vi "T1T2占空比.vi"() -> ()   [LabVIEW 2020]
uses:
  <vilib>/DAQmx/read.llb/DAQmx Read (Counter 1D DBL 1Chan NSamp).vi
  Global_Variable/Global.vi
  <vilib>/DAQmx/create/channels.llb/DAQmx Create Channel (CI-Period).vi
  <vilib>/DAQmx/configure/timing.llb/DAQmx Timing (Implicit).vi
  <vilib>/DAQmx/miscellaneous.llb/DAQmx Fill In Error Info.vi
  <userlib>/_MGI/1D Array/MGI Average/MGI Average (DBL[]).vi
  <vilib>/DAQmx/create/channels.llb/DAQmx Create Channel (CI-Pulse Width).vi
  <resource>/objmgr/daqmx.rc
panel:
  out "T1 2":dbl
  out "T2 2":dbl
  out "T2":dbl
  out "T2周期":dbl
  out "T1周期":dbl
  out "T1":dbl
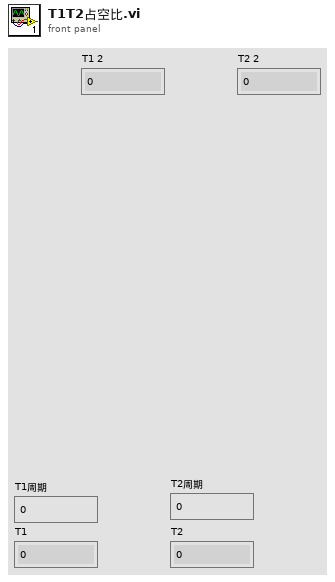
[diagram p1: front panel]
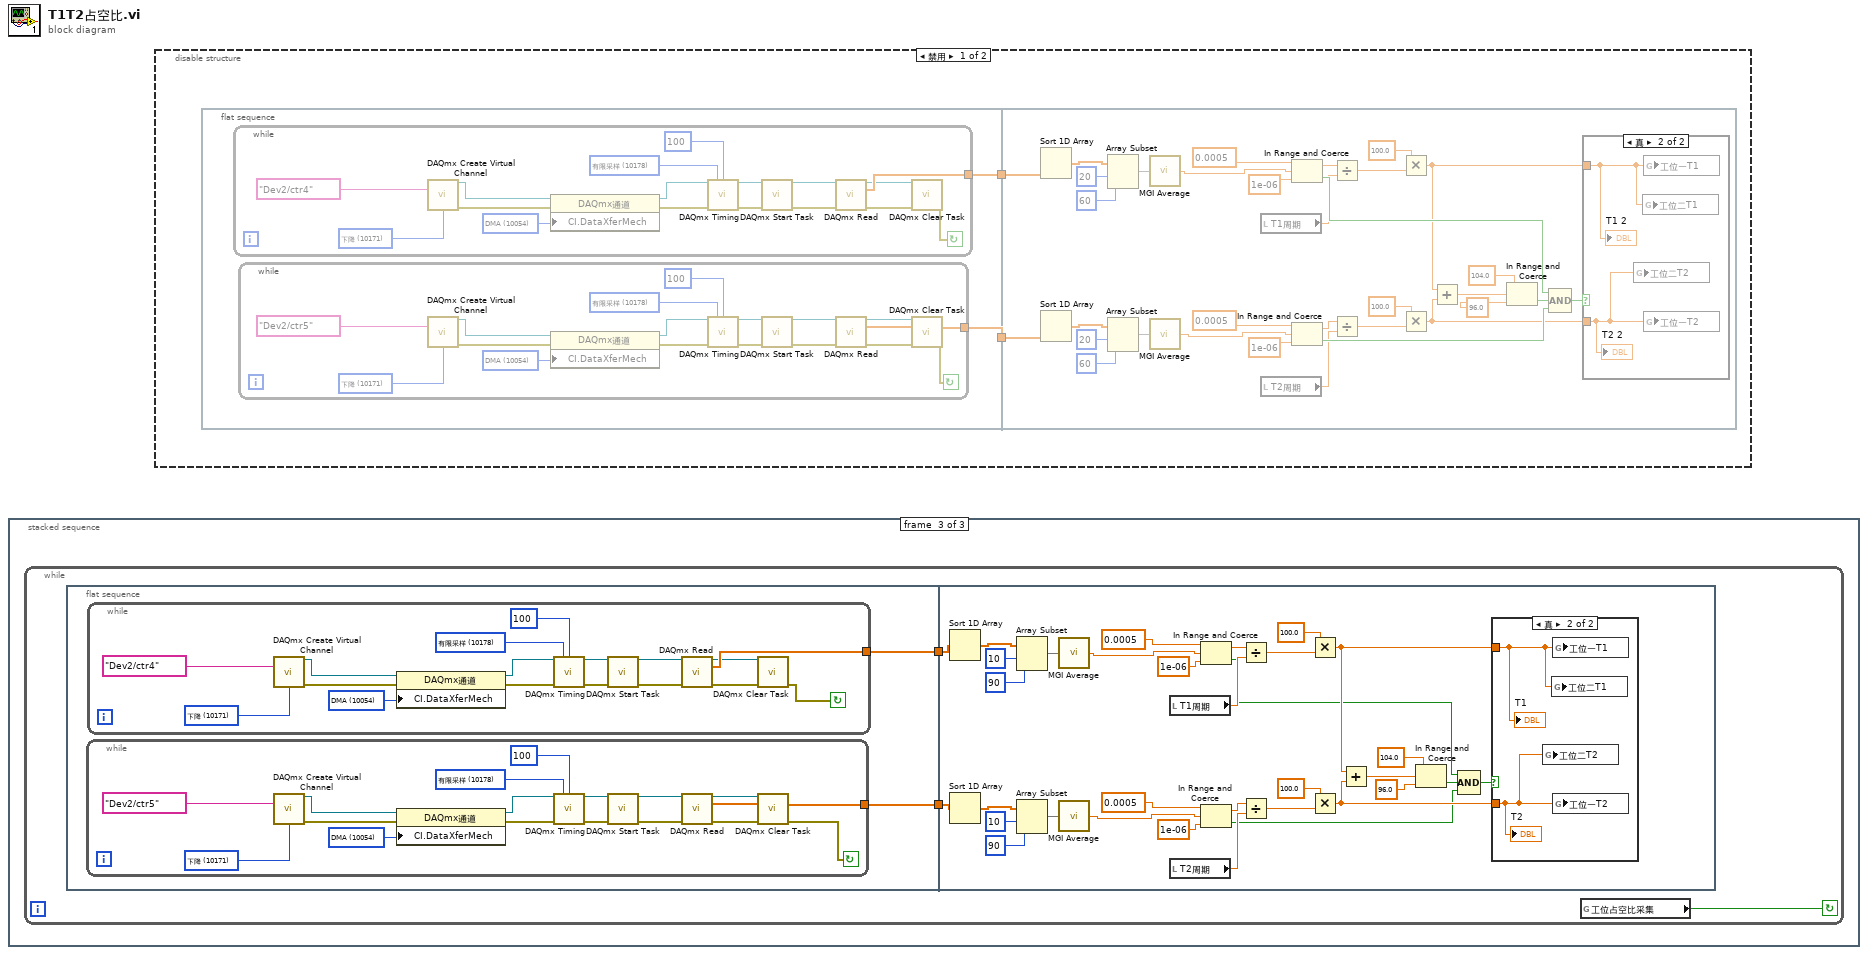
[diagram p0: block diagram]
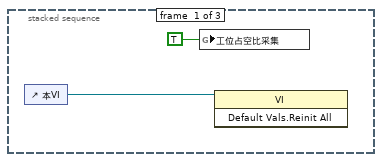
[diagram p4: hidden frame]
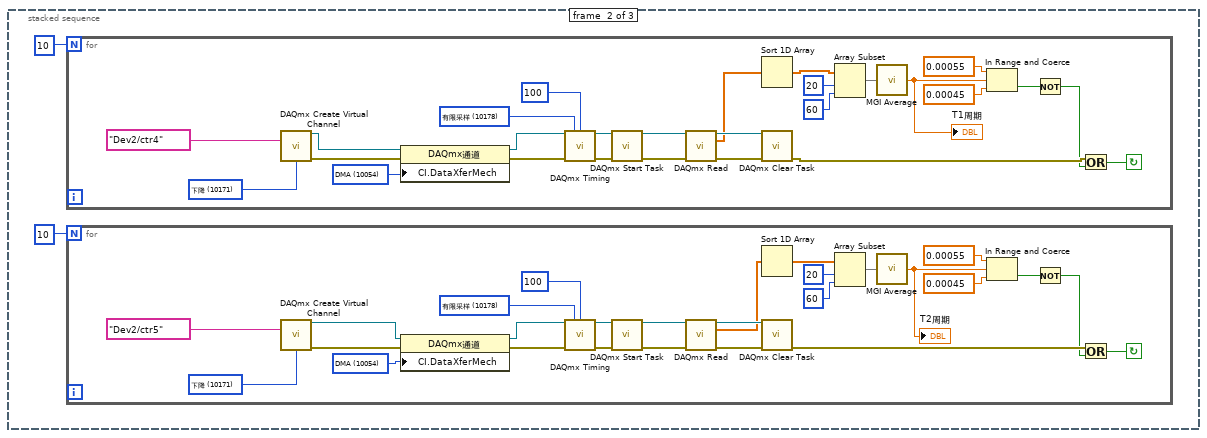
[diagram p5: hidden frame]
diagram:
  n1 = stacked-sequence {
    frame #0 {
      n2 = control-ref of="本VI"() -> (w2:refnum<vi>)
      n3 = global write "Global.vi" "工位占空比采集"(TRUE ("工位一占空比采集")) -> ()
      n4 = invoke class="VI" method="Default Vals.Reinit All"(reference=w2) -> ()  [unwired: 2 in, 3 out]
    }
    frame #1 {
      n5 = for {
        N: 10 -> [_]
        stop <- w32 continue-if-true
        w45 = 10054 items=["DMA"=10054, "中断"=10204, "程序控制I/O"=10264, "USB Bulk"=12590] ("CI.DataXferMech")
        w49 = 10178 items=["有限采样"=10178, "连续采样"=10123, "硬件定时单点"=12522] ("sample mode")
        w58 = 10171 items=["上升"=10280, "下降"=10171] ("starting edge")
        n6 = call-poly <vilib>:"DAQmx Create Virtual Channel.vi"("counter"=tag "Dev2/ctr4", "starting edge"=w58) -> ("task out"=w57:refnum<k21>, "error out"=w47:errorcluster)  [unwired: 12 in]
        n7 = property class="DAQmx通道"(reference=w57, error in=w47, "CI.DataXferMech"=w45) -> (reference out=w48:refnum<k21>, error out=w46:errorcluster)
        n8 = call-poly <vilib>:"DAQmx Timing.vi"("task/channels in"=w48, "sample mode"=w49, "samples per channel"=100, "error in"=w46) -> ("task out"=w56:refnum<k21>, "error out"=w55:errorcluster)  [unwired: 10 in]
        n9 = call <vilib>:"DAQmx Start Task.vi"("task/channels in"=w56, "error in"=w55) -> ("task out"=w54:refnum<k21>, "error out"=w53:errorcluster)  [unwired: 12 in]
        n10 = call-poly <vilib>:"DAQmx Read.vi"("task/channels in"=w54, "error in"=w53) -> ("task out"=w51:refnum<k21>, "data"=w39:dbl[], "error out"=w52:errorcluster)  [unwired: 11 in]
        n11 = Sort 1D Array(array=w39) -> (sorted array=w42:dbl[])
        n12 = call <vilib>:"DAQmx Clear Task.vi"("task in"=w51, "error in"=w52) -> ("error out"=w34:errorcluster)  [unwired: 13 in]
        n13 = Array Subset(array=w42, index=20 ("索引"), length=60 ("长度")) -> (w43:dbl[])
        n14 = call-poly <userlib>:"MGI Average.vi"("Double[]"=w43) -> ("Average"=w38:dbl)  [unwired: 1 in]
        "T1周期" <- w38
        n15 = In Range and Coerce(upper limit=0.00055 ("上限"), x=w38, lower limit=0.00045 ("上限")) -> (In Range?=w35:bool)  [unwired: 1 out]
        n16 = Not(x=w35) -> (.not. x?=w33:bool)
        n17 = Or(x=w34, y=w33) -> (x .or. y?=w32:bool)
      }
      n18 = for {
        N: 10 -> [_]
        stop <- w5 continue-if-true
        w18 = 10054 items=["DMA"=10054, "中断"=10204, "程序控制I/O"=10264, "USB Bulk"=12590] ("CI.DataXferMech")
        w22 = 10178 items=["有限采样"=10178, "连续采样"=10123, "硬件定时单点"=12522] ("sample mode")
        w31 = 10171 items=["上升"=10280, "下降"=10171] ("starting edge")
        n19 = call-poly <vilib>:"DAQmx Create Virtual Channel.vi"("counter"=tag "Dev2/ctr5", "starting edge"=w31) -> ("task out"=w30:refnum<k21>, "error out"=w20:errorcluster)  [unwired: 12 in]
        n20 = property class="DAQmx通道"(reference=w30, error in=w20, "CI.DataXferMech"=w18) -> (reference out=w21:refnum<k21>, error out=w19:errorcluster)
        n21 = call-poly <vilib>:"DAQmx Timing.vi"("task/channels in"=w21, "sample mode"=w22, "samples per channel"=100, "error in"=w19) -> ("task out"=w29:refnum<k21>, "error out"=w28:errorcluster)  [unwired: 10 in]
        n22 = call <vilib>:"DAQmx Start Task.vi"("task/channels in"=w29, "error in"=w28) -> ("task out"=w27:refnum<k21>, "error out"=w26:errorcluster)  [unwired: 12 in]
        n23 = call-poly <vilib>:"DAQmx Read.vi"("task/channels in"=w27, "error in"=w26) -> ("task out"=w24:refnum<k21>, "data"=w12:dbl[], "error out"=w25:errorcluster)  [unwired: 11 in]
        n24 = Sort 1D Array(array=w12) -> (sorted array=w16:dbl[])
        n25 = call <vilib>:"DAQmx Clear Task.vi"("task in"=w24, "error in"=w25) -> ("error out"=w8:errorcluster)  [unwired: 13 in]
        n26 = Array Subset(array=w16, index=20 ("索引"), length=60 ("长度")) -> (w15:dbl[])
        n27 = call-poly <userlib>:"MGI Average.vi"("Double[]"=w15) -> ("Average"=w9:dbl)  [unwired: 1 in]
        "T2周期" <- w9
        n28 = In Range and Coerce(upper limit=0.00055 ("上限"), x=w9, lower limit=0.00045 ("上限")) -> (In Range?=w7:bool)  [unwired: 1 out]
        n29 = Not(x=w7) -> (.not. x?=w6:bool)
        n30 = Or(x=w8, y=w6) -> (x .or. y?=w5:bool)
      }
    }
    frame #2 {
      n31 = while {
        stop <- w61 continue-if-true
        n32 = flat-sequence {
          tunnel: [w63] -> w60
          tunnel: [w62] -> w59
          tunnel: w60 -> [w98]
          tunnel: w59 -> [w101]
          frame #0 {
            n33 = while {
              tunnel: [w80] -> w62
              stop <- w64 continue-if-true
              w66 = 10054 items=["DMA"=10054, "中断"=10204, "程序控制I/O"=10264, "USB Bulk"=12590] ("CI.DataXferMech")
              w70 = 10178 items=["有限采样"=10178, "连续采样"=10123, "硬件定时单点"=12522] ("sample mode")
              w79 = 10171 items=["上升"=10280, "下降"=10171] ("starting edge")
              n34 = call-poly <vilib>:"DAQmx Create Virtual Channel.vi"("counter"=tag "Dev2/ctr5", "starting edge"=w79) -> ("task out"=w78:refnum<k21>, "error out"=w68:errorcluster)  [unwired: 12 in]
              n35 = property class="DAQmx通道"(reference=w78, error in=w68, "CI.DataXferMech"=w66) -> (reference out=w69:refnum<k21>, error out=w67:errorcluster)
              n36 = call-poly <vilib>:"DAQmx Timing.vi"("task/channels in"=w69, "sample mode"=w70, "samples per channel"=100, "error in"=w67) -> ("task out"=w77:refnum<k21>, "error out"=w76:errorcluster)  [unwired: 10 in]
              n37 = call <vilib>:"DAQmx Start Task.vi"("task/channels in"=w77, "error in"=w76) -> ("task out"=w75:refnum<k21>, "error out"=w74:errorcluster)  [unwired: 12 in]
              n38 = call-poly <vilib>:"DAQmx Read.vi"("task/channels in"=w75, "error in"=w74) -> ("task out"=w72:refnum<k21>, "data"=w80:dbl[], "error out"=w73:errorcluster)  [unwired: 11 in]
              n39 = call <vilib>:"DAQmx Clear Task.vi"("task in"=w72, "error in"=w73) -> ("error out"=w64:errorcluster)  [unwired: 13 in]
            }
            n40 = while {
              tunnel: [w97] -> w63
              stop <- w81 continue-if-true
              w83 = 10054 items=["DMA"=10054, "中断"=10204, "程序控制I/O"=10264, "USB Bulk"=12590] ("CI.DataXferMech")
              w87 = 10178 items=["有限采样"=10178, "连续采样"=10123, "硬件定时单点"=12522] ("sample mode")
              w96 = 10171 items=["上升"=10280, "下降"=10171] ("starting edge")
              n41 = call-poly <vilib>:"DAQmx Create Virtual Channel.vi"("counter"=tag "Dev2/ctr4", "starting edge"=w96) -> ("task out"=w95:refnum<k21>, "error out"=w85:errorcluster)  [unwired: 12 in]
              n42 = property class="DAQmx通道"(reference=w95, error in=w85, "CI.DataXferMech"=w83) -> (reference out=w86:refnum<k21>, error out=w84:errorcluster)
              n43 = call-poly <vilib>:"DAQmx Timing.vi"("task/channels in"=w86, "sample mode"=w87, "samples per channel"=100, "error in"=w84) -> ("task out"=w94:refnum<k21>, "error out"=w93:errorcluster)  [unwired: 10 in]
              n44 = call <vilib>:"DAQmx Start Task.vi"("task/channels in"=w94, "error in"=w93) -> ("task out"=w92:refnum<k21>, "error out"=w91:errorcluster)  [unwired: 12 in]
              n45 = call-poly <vilib>:"DAQmx Read.vi"("task/channels in"=w92, "error in"=w91) -> ("task out"=w89:refnum<k21>, "data"=w97:dbl[], "error out"=w90:errorcluster)  [unwired: 11 in]
              n46 = call <vilib>:"DAQmx Clear Task.vi"("task in"=w89, "error in"=w90) -> ("error out"=w81:errorcluster)  [unwired: 13 in]
            }
          }
          frame #1 {
            n47 = Sort 1D Array(array=w98) -> (sorted array=w130:dbl[])
            n48 = Sort 1D Array(array=w101) -> (sorted array=w127:dbl[])
            n49 = Array Subset(array=w130, index=10 ("索引"), length=90 ("长度")) -> (w129:dbl[])
            n50 = Array Subset(array=w127, index=10 ("索引"), length=90 ("长度")) -> (w128:dbl[])
            n51 = call-poly <userlib>:"MGI Average.vi"("Double[]"=w129) -> ("Average"=w126:dbl)  [unwired: 1 in]
            n52 = call-poly <userlib>:"MGI Average.vi"("Double[]"=w128) -> ("Average"=w124:dbl)  [unwired: 1 in]
            n53 = local read "T1周期"() -> (w121:dbl)
            n54 = local read "T2周期"() -> (w120:dbl)
            n55 = In Range and Coerce(upper limit=0.0005 ("上限"), x=w126, lower limit=1e-06 ("上限")) -> (coerced(x)=w125:dbl, In Range?=w115:bool)
            n56 = In Range and Coerce(upper limit=0.0005 ("上限"), x=w124, lower limit=1e-06 ("上限")) -> (coerced(x)=w123:dbl, In Range?=w114:bool)
            n57 = Divide(x=w125, y=w121) -> (x/y=w122:dbl)
            n58 = Divide(x=w123, y=w120) -> (x/y=w119:dbl)
            n59 = Multiply(x=100.0, y=w122) -> (x*y=w118:dbl)
            n60 = Multiply(x=100.0, y=w119) -> (x*y=w117:dbl)
            n61 = Add(x=w118, y=w117) -> (x+y=w116:dbl)
            n62 = In Range and Coerce(upper limit=104.0 ("上限"), x=w116, lower limit=96.0 ("下限")) -> (In Range?=w113:bool)  [unwired: 1 out]
            n63 = Compound Arithmetic op=AND ("复合运算")(w115, w113, w114) -> (w112:bool)
            n64 = case shown="真" w112 {
              tunnel: w118 -> [_ w132]
              tunnel: w117 -> [_ w131]
              frame False {
              }
              frame True {
                n65 = global write "Global.vi" "工位二T2"(w131) -> ()
                n66 = global write "Global.vi" "工位二T1"(w132) -> ()
                n67 = global write "Global.vi" "工位一T1"(w132) -> ()
                n68 = global write "Global.vi" "工位一T2"(w131) -> ()
                "T1" <- w132
                "T2" <- w131
              }
            }
          }
        }
        n69 = global read "Global.vi" "工位占空比采集"() -> (w61:bool)
      }
    }
  }
  n70 = disable-structure shown="禁用" {
    frame Disabled {
      n71 = flat-sequence {
        tunnel: [w136] -> w134
        tunnel: [w135] -> w133
        tunnel: w134 -> [w171]
        tunnel: w133 -> [w174]
        frame #0 {
          n72 = while {
            tunnel: [w170] -> w136
            stop <- w154 continue-if-true
            w156 = 10054 items=["DMA"=10054, "中断"=10204, "程序控制I/O"=10264, "USB Bulk"=12590] ("CI.DataXferMech")
            w160 = 10178 items=["有限采样"=10178, "连续采样"=10123, "硬件定时单点"=12522] ("sample mode")
            w169 = 10171 items=["上升"=10280, "下降"=10171] ("starting edge")
            n73 = call-poly <vilib>:"DAQmx Create Virtual Channel.vi"("counter"=tag "Dev2/ctr4", "starting edge"=w169) -> ("task out"=w168:refnum<k21>, "error out"=w158:errorcluster)  [unwired: 12 in]
            n74 = property class="DAQmx通道"(reference=w168, error in=w158, "CI.DataXferMech"=w156) -> (reference out=w159:refnum<k21>, error out=w157:errorcluster)
            n75 = call-poly <vilib>:"DAQmx Timing.vi"("task/channels in"=w159, "sample mode"=w160, "samples per channel"=100, "error in"=w157) -> ("task out"=w167:refnum<k21>, "error out"=w166:errorcluster)  [unwired: 10 in]
            n76 = call <vilib>:"DAQmx Start Task.vi"("task/channels in"=w167, "error in"=w166) -> ("task out"=w165:refnum<k21>, "error out"=w164:errorcluster)  [unwired: 12 in]
            n77 = call-poly <vilib>:"DAQmx Read.vi"("task/channels in"=w165, "error in"=w164) -> ("task out"=w162:refnum<k21>, "data"=w170:dbl[], "error out"=w163:errorcluster)  [unwired: 11 in]
            n78 = call <vilib>:"DAQmx Clear Task.vi"("task in"=w162, "error in"=w163) -> ("error out"=w154:errorcluster)  [unwired: 13 in]
          }
          n79 = while {
            tunnel: [w153] -> w135
            stop <- w137 continue-if-true
            w139 = 10054 items=["DMA"=10054, "中断"=10204, "程序控制I/O"=10264, "USB Bulk"=12590] ("CI.DataXferMech")
            w143 = 10178 items=["有限采样"=10178, "连续采样"=10123, "硬件定时单点"=12522] ("sample mode")
            w152 = 10171 items=["上升"=10280, "下降"=10171] ("starting edge")
            n80 = call-poly <vilib>:"DAQmx Create Virtual Channel.vi"("counter"=tag "Dev2/ctr5", "starting edge"=w152) -> ("task out"=w151:refnum<k21>, "error out"=w141:errorcluster)  [unwired: 12 in]
            n81 = property class="DAQmx通道"(reference=w151, error in=w141, "CI.DataXferMech"=w139) -> (reference out=w142:refnum<k21>, error out=w140:errorcluster)
            n82 = call-poly <vilib>:"DAQmx Timing.vi"("task/channels in"=w142, "sample mode"=w143, "samples per channel"=100, "error in"=w140) -> ("task out"=w150:refnum<k21>, "error out"=w149:errorcluster)  [unwired: 10 in]
            n83 = call <vilib>:"DAQmx Start Task.vi"("task/channels in"=w150, "error in"=w149) -> ("task out"=w148:refnum<k21>, "error out"=w147:errorcluster)  [unwired: 12 in]
            n84 = call-poly <vilib>:"DAQmx Read.vi"("task/channels in"=w148, "error in"=w147) -> ("task out"=w145:refnum<k21>, "data"=w153:dbl[], "error out"=w146:errorcluster)  [unwired: 11 in]
            n85 = call <vilib>:"DAQmx Clear Task.vi"("task in"=w145, "error in"=w146) -> ("error out"=w137:errorcluster)  [unwired: 13 in]
          }
        }
        frame #1 {
          n86 = Sort 1D Array(array=w171) -> (sorted array=w185:dbl[])
          n87 = Sort 1D Array(array=w174) -> (sorted array=w188:dbl[])
          n88 = Array Subset(array=w185, index=20 ("索引"), length=60 ("长度")) -> (w186:dbl[])
          n89 = Array Subset(array=w188, index=20 ("索引"), length=60 ("长度")) -> (w187:dbl[])
          n90 = call-poly <userlib>:"MGI Average.vi"("Double[]"=w186) -> ("Average"=w189:dbl)  [unwired: 1 in]
          n91 = call-poly <userlib>:"MGI Average.vi"("Double[]"=w187) -> ("Average"=w191:dbl)  [unwired: 1 in]
          n92 = local read "T1周期"() -> (w194:dbl)
          n93 = local read "T2周期"() -> (w195:dbl)
          n94 = In Range and Coerce(upper limit=0.0005 ("上限"), x=w189, lower limit=1e-06 ("上限")) -> (coerced(x)=w190:dbl, In Range?=w200:bool)
          n95 = In Range and Coerce(upper limit=0.0005 ("上限"), x=w191, lower limit=1e-06 ("上限")) -> (coerced(x)=w192:dbl, In Range?=w201:bool)
          n96 = Divide(x=w190, y=w194) -> (x/y=w193:dbl)
          n97 = Divide(x=w192, y=w195) -> (x/y=w196:dbl)
          n98 = Multiply(x=100.0, y=w193) -> (x*y=w197:dbl)
          n99 = Multiply(x=100.0, y=w196) -> (x*y=w198:dbl)
          n100 = Add(x=w197, y=w198) -> (x+y=w199:dbl)
          n101 = In Range and Coerce(upper limit=104.0 ("上限"), x=w199, lower limit=96.0 ("下限")) -> (In Range?=w202:bool)  [unwired: 1 out]
          n102 = Compound Arithmetic op=AND ("复合运算")(w200, w202, w201) -> (w203:bool)
          n103 = case shown="真" w203 {
            tunnel: w197 -> [_ w205]
            tunnel: w198 -> [_ w204]
            frame False {
            }
            frame True {
              n104 = global write "Global.vi" "工位二T2"(w204) -> ()
              n105 = global write "Global.vi" "工位二T1"(w205) -> ()
              n106 = global write "Global.vi" "工位一T1"(w205) -> ()
              n107 = global write "Global.vi" "工位一T2"(w204) -> ()
              "T1 2" <- w205
              "T2 2" <- w204
            }
          }
        }
      }
    }
    frame Enabled {
    }
  }
